vi "CC_Load_Test_REV2.vi"() -> ()   [LabVIEW 2018]
uses:
  <vilib>/Utility/error.llb/DialogType.ctl
  <vilib>/DAQmx/read.llb/DAQmx Read (Analog 1D Wfm NChan NSamp).vi
  <vilib>/Waveform/WDTOps.llb/WDT Get Waveform Time Array DBL.vi
  <vilib>/DAQmx/configure/timing.llb/DAQmx Timing (Sample Clock).vi
  <vilib>/DAQmx/miscellaneous.llb/DAQmx Fill In Error Info.vi
  <resource>/objmgr/daqmx.rc
panel:
  out "Strain Gauges":waveform(dbl)[](graph) caption="Waveform Chart"
  in  "Tab Control":enum32{"Telemetry", "DAQ Settings"}(tab)
  in  "Save 2":bool caption="Save"
  out "Save Path":path caption="Path"
  in  "Test Name":string caption="String"
  in  "Stop 4":bool caption="Stop"
  in  "Strain Tare":bool caption="Reset"
  out "Strain 0":dbl caption="Numeric" format="%#_3e"
  out "Strain 1":dbl caption="Numeric" format="%#_3e"
  out "Strain 2":dbl caption="Numeric" format="%#_3e"
  out "Strain 3":dbl caption="Numeric" format="%#_3e"
  out "Strain 4":dbl caption="Numeric" format="%#_3e"
  out "Strain 5":dbl caption="Numeric" format="%#_3e"
  out "Strain 6":dbl caption="Numeric" format="%#_3e"
  out "Strain 7":dbl caption="Numeric" format="%#_3e"
  out "Strain 8":dbl caption="Numeric" format="%#_3e"
  out "Strain 9":dbl caption="Numeric" format="%#_3e"
  out "Strain 10":dbl caption="Numeric" format="%#_3e"
  out "Strain 11":dbl caption="Numeric" format="%#_3e"
  out "Strain 12":dbl caption="Numeric" format="%#_3e"
  out "Strain 13":dbl caption="Numeric" format="%#_3e"
  out "Strain 14":dbl caption="Numeric" format="%#_3e"
  out "Strain 15":dbl caption="Numeric" format="%#_3e"
  out "LOAD":dbl caption="Numeric"
  out "LOAD 2":dbl caption="Numeric"
  in  "Load Tare":bool caption="Reset"
  in  "Strain Samples Per Loop":i32=100 caption="Numeric"
  out "Strain Output Rate":dbl caption="Numeric"
  in  "Strain Sample Rate":dbl=1000.0 caption="Numeric"
  out "Load Cell Output Rate":dbl caption="Numeric"
  in  "Load Cell Sample Rate":dbl=100.0 caption="Numeric"
  in  "Load Cell Samples Per Loop":i32=10 caption="Numeric"
  out "Load Cell":waveform(dbl)[](graph) caption="Waveform Chart"
  # "Raw"
  # "Tared"
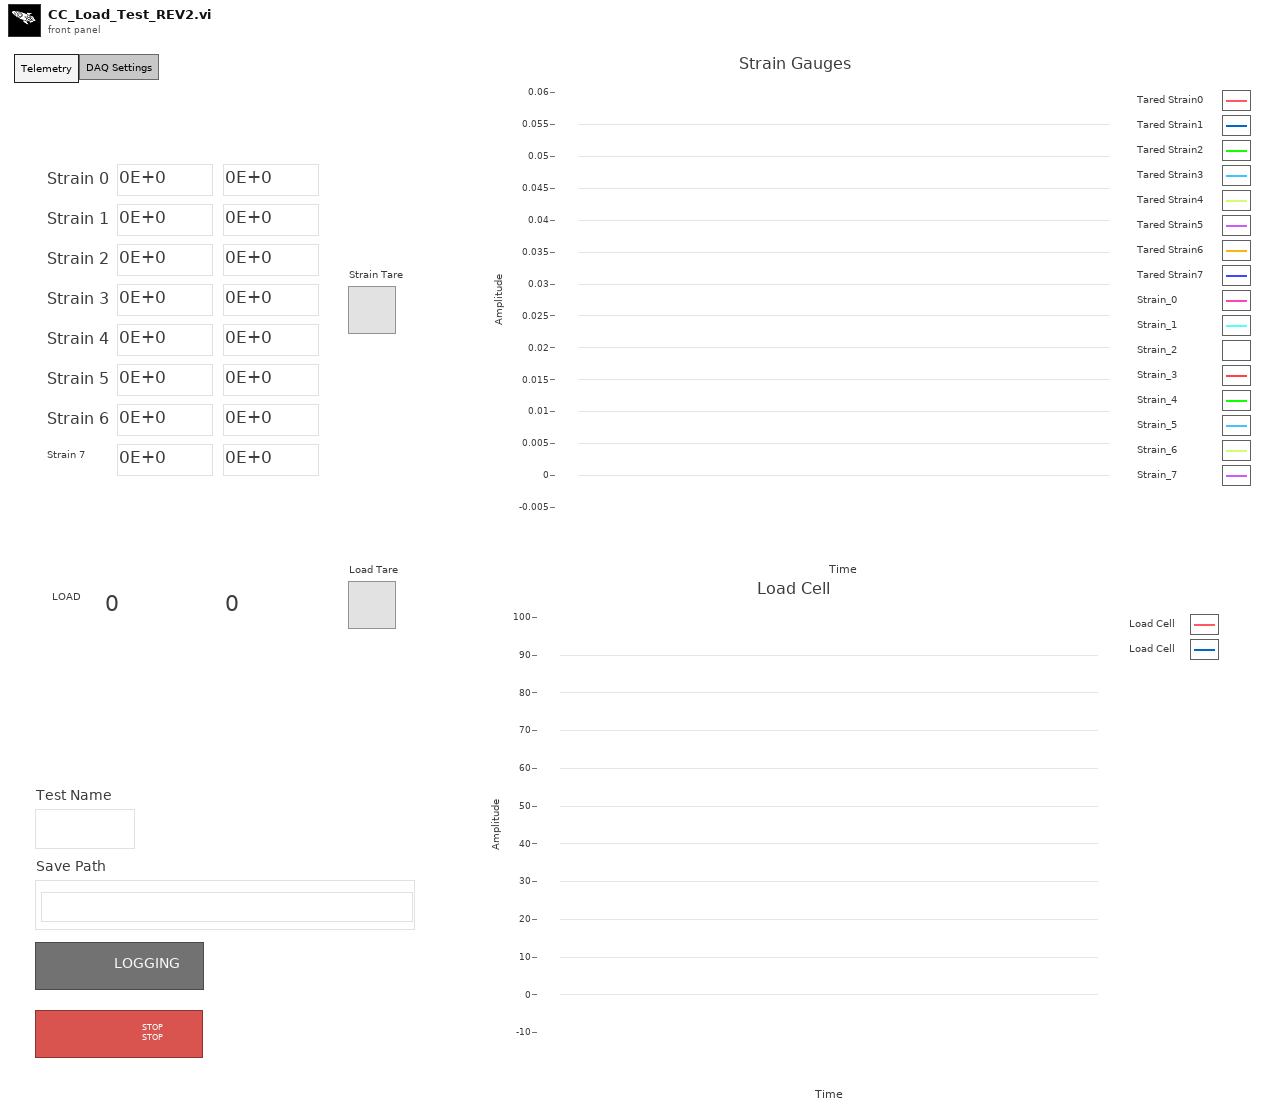
[diagram p1: front panel]
types:
  T1 = typedef "DialogType.ctl" = u16
  T2 = enum16{"open", "open or create", "create or replace", "create", "open (read-only)"}
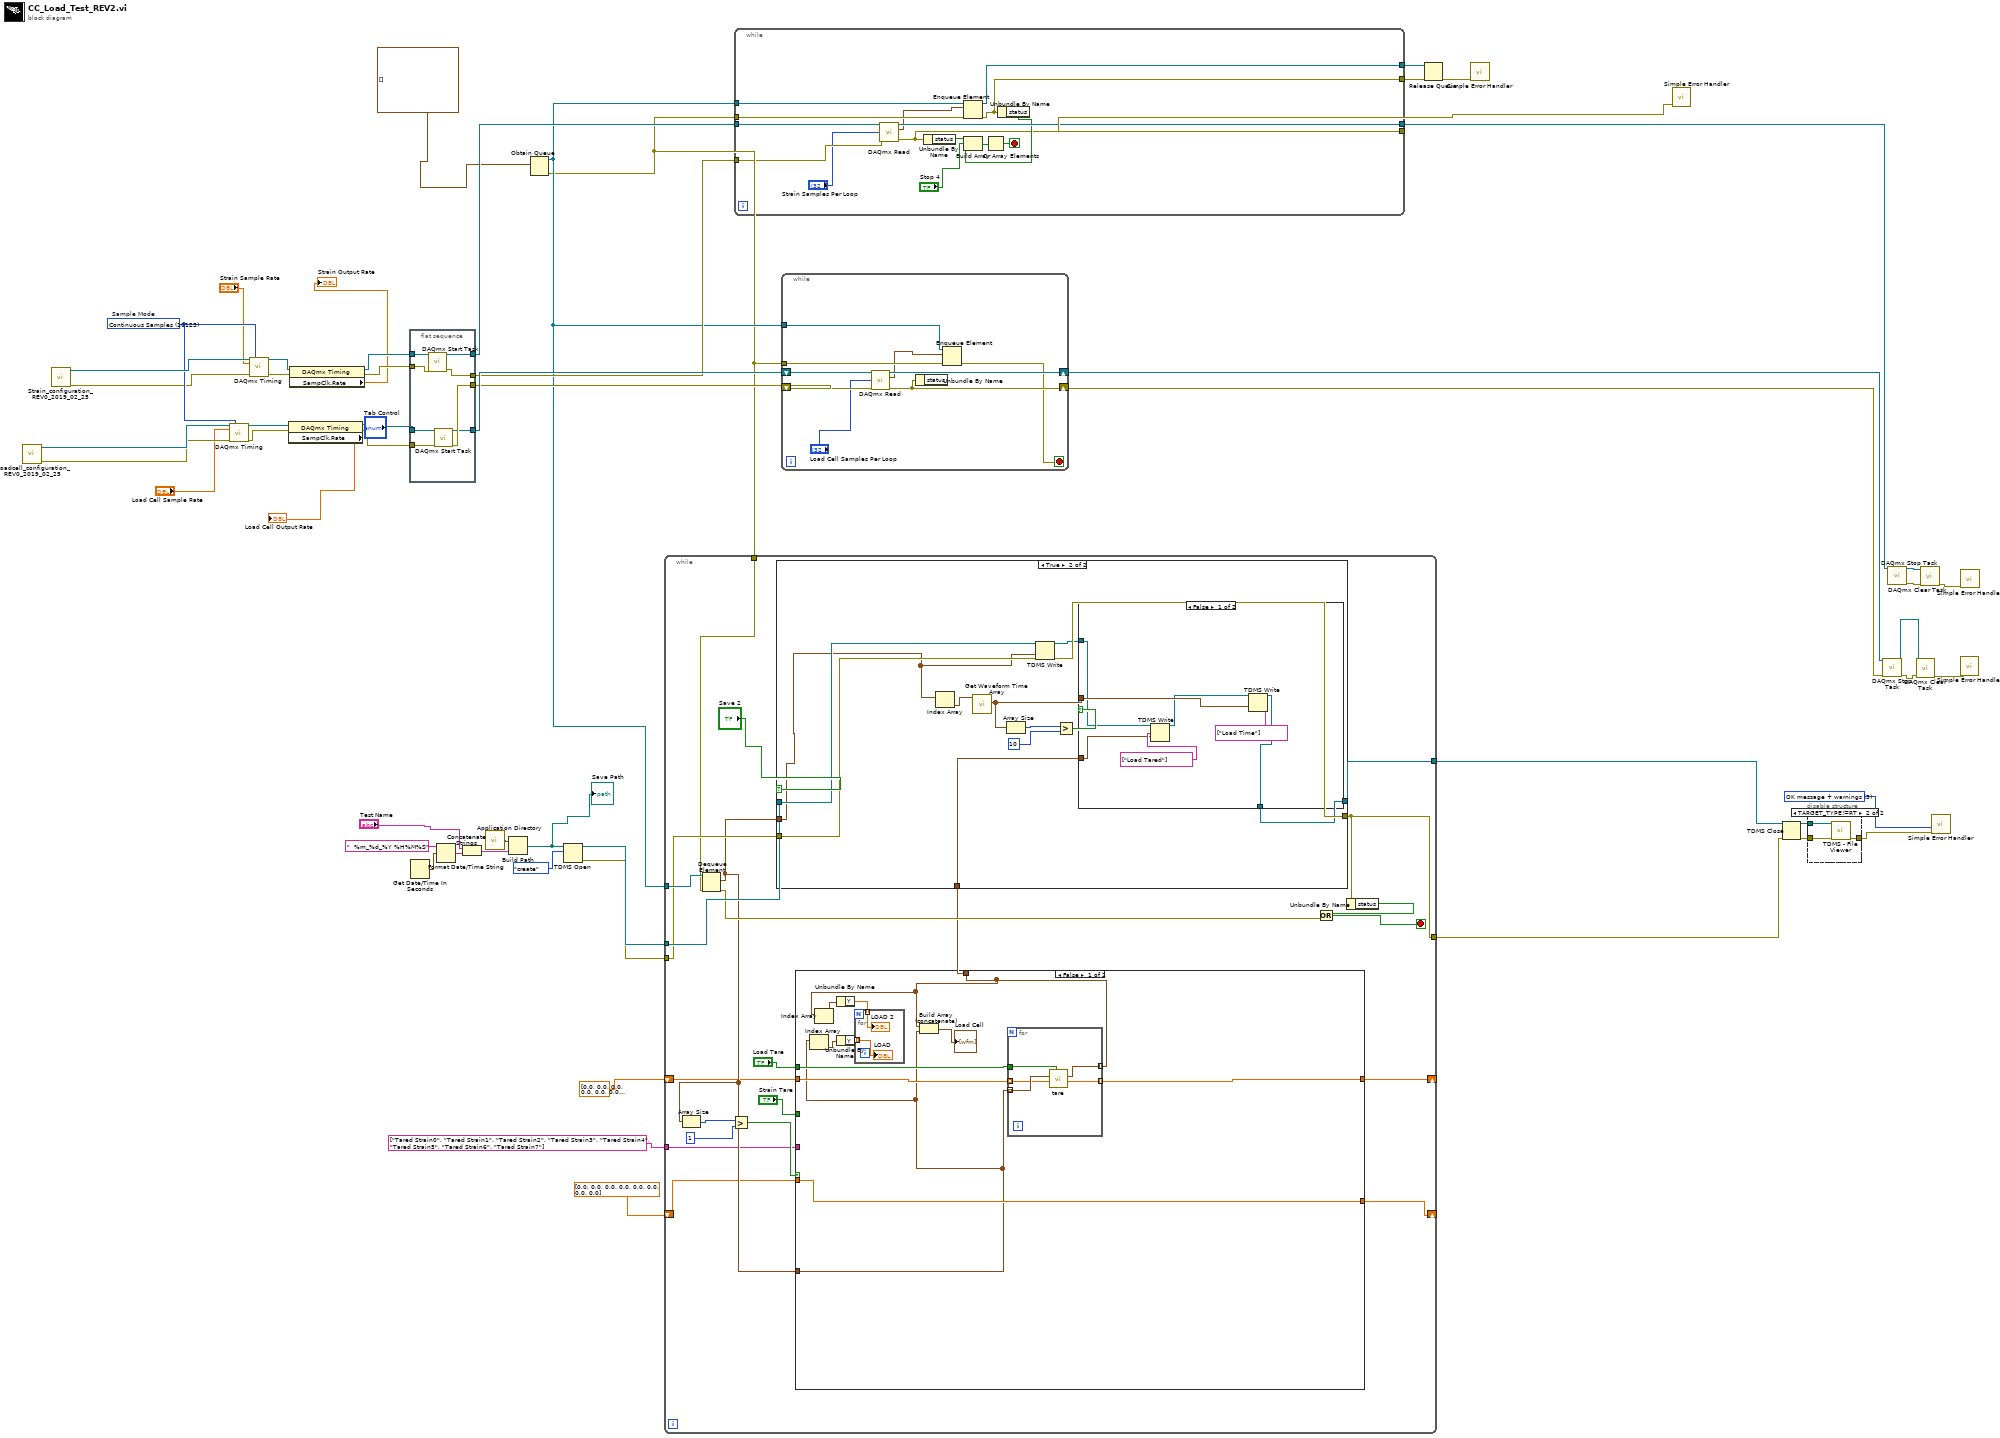
[diagram p0: block diagram]
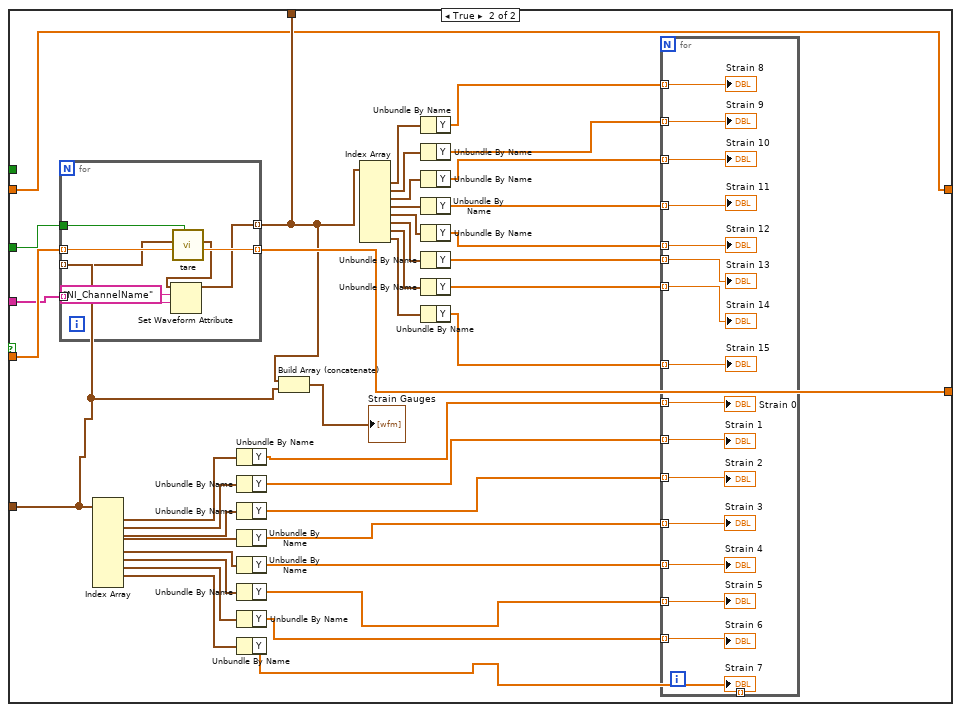
[diagram p3: hidden frame]
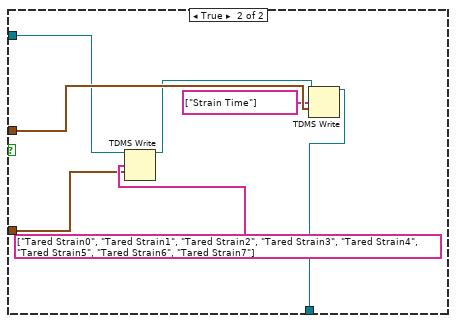
[diagram p5: hidden frame]
diagram:
  w47 = T1 3 items=["no dialog", "OK message", "continue or stop message", "OK message + warnings", "continue/stop + warnings"] ("type of dialog (OK msg:1)")
  w34 = 10123 items=["Finite Samples"=10178, "Continuous Samples"=10123, "Hardware Timed Single Point"=12522]  # Sample Mode
  n1 = call "Loadcell_configuration_REV0_2019_02_25.vi"() -> ("error out"=w24:errorcluster, "task out"=w31:refnum<k21>)  [unwired: 10 in]
  n2 = call "Strain_configuration_REV0_2019_02_25.vi"() -> ("error out"=w25:errorcluster, "task out"=w35:refnum<k21>)  [unwired: 10 in]
  n3 = call-poly <vilib>:"DAQmx Timing.vi"("task/channels in"=w31, "sample mode"=w34, "rate"="Load Cell Sample Rate", "error in"=w24) -> ("task out"=w33:refnum<k21>, "error out"=w32:errorcluster)  [unwired: 10 in]
  n4 = call-poly <vilib>:"DAQmx Timing.vi"("task/channels in"=w35, "sample mode"=w34, "rate"="Strain Sample Rate", "error in"=w25) -> ("task out"=w56:refnum<k21>, "error out"=w55:errorcluster)  [unwired: 10 in]
  n5 = property class="DAQmx Timing"(reference=w33, error in=w32) -> (reference out=w30:refnum<k21>, error out=w22:errorcluster, "SampClk.Rate"=→"Load Cell Output Rate":dbl)
  n6 = property class="DAQmx Timing"(reference=w56, error in=w55) -> (reference out=w50:refnum<k21>, error out=w49:errorcluster, "SampClk.Rate"=→"Strain Output Rate":dbl)
  n7 = flat-sequence {
    tunnel: [w64] -> w54
    tunnel: w50 -> [w63]
    tunnel: w49 -> [w62]
    tunnel: [w61] -> w18
    tunnel: w30 -> [w60]
    tunnel: [w59] -> w17
    tunnel: [w58] -> w20
    tunnel: w22 -> [w57]
    frame #0 {
      n8 = call <vilib>:"DAQmx Start Task.vi"("task/channels in"=w63, "error in"=w62) -> ("task out"=w64:refnum<k21>, "error out"=w61:errorcluster)  [unwired: 12 in]
      n9 = call <vilib>:"DAQmx Start Task.vi"("task/channels in"=w60, "error in"=w57) -> ("task out"=w58:refnum<k21>, "error out"=w59:errorcluster)  [unwired: 12 in]
    }
  }
  n10 = Get Date/Time In Seconds() -> (seconds since 1Jan1904=w40:timestamp)
  n11 = Format Date/Time String(time format string (%c)="  %m_%d_%Y %H%M%S", seconds (now)=w40) -> (date/time string=w37:string)  [unwired: 1 in]
  n12 = Concatenate Strings("Test Name", w37) -> (w36:string)
  n13 = call <vilib>:"Application Directory.vi"() -> ("Application Directory"=w38:path)
  n14 = Build Path(base path=w38, name or relative path=w36) -> (appended path=w5:path)
  "Save Path" <- w5
  n15 = Obtain Queue(element data type=waveform(dbl)[] [] ("data")) -> (queue out=w16:refnum<queue>, error out=w10:errorcluster)  [unwired: 4 in, 1 out]
  n16 = TDMS Open(10:T2."create" ("operation"), 11:w5) -> (0:w41:errorcluster, 3:w46:refnum<k34>)  [unwired: 5 in]
  n17 = while {
    tunnel: w46 -> [w86]
    tunnel: [w85] -> w45
    tunnel: [w82] -> w42
    tunnel: w41 -> [w80]
    tunnel: w16 -> [w81]
    tunnel: w10 -> [w79]
    shift-right: [w70] -> _
    shift-left: dbl[] [0.0, 0.0, 0.0, 0.0, 0.0, 0.0, 0.0, 0.0] ("Shift Registor") -> [w71]
    shift-right: [w67] -> _
    shift-left: dbl[] [0.0, 0.0, 0.0, 0.0, 0.0, 0.0, 0.0, 0.0] ("Shift Registor") -> [w68]
    tunnel: string[] ["Tared Strain0", "Tared Strain1", "Tared Strain2", "Tared Strain3", "Tared Strain4", "Tared Strain5", "Tared Strain6", "Tared Strain7"] ("channel name(s) in (Untitled)") -> [w66]
    stop <- w83 stop-if-true
    n18 = Dequeue Element(queue=w81, error in (no error)=w79) -> (element=w72:waveform(dbl)[], error out=w78:errorcluster)  [unwired: 1 in, 2 out]
    n19 = Array Size(array=w72) -> (size(s)=w75:i32)
    n20 = Greater?(x=w75, y=1) -> (0:w73:bool)
    n21 = case shown="False" w73 {
      tunnel: "Strain Tare" -> [_ w110]
      tunnel: w71 -> [w97 w112]
      tunnel: w72 -> [w89 w109]
      tunnel: [w97 w111] -> w70
      tunnel: [w93 w108] -> w69
      tunnel: w68 -> [w96 w106]
      tunnel: [w95 w106] -> w67
      tunnel: w66 -> [_ w105]
      tunnel: "Load Tare" -> [w90 _]
      frame False {
        n22 = Index Array(array=w89) -> (element=w88:waveform(dbl))  [unwired: 1 in]
        n23 = Unbundle By Name(w88) -> ("Y"=w87:dbl[])
        n24 = for {
          tunnel: w89 -> [w102] mode=indexing
          tunnel: w96 -> [w101] mode=indexing
          tunnel: [w100] -> w95 mode=indexing
          tunnel: [w104] -> w93 mode=indexing
          tunnel: w90 -> [w103]
          n25 = call "tare.vi"("Tare Control"=w103, "Shift Registor"=w101, "Input Waveform"=w102) -> ("Shift Registor Out"=w100:dbl, "output waveform"=w104:waveform(dbl))  [unwired: 7 in]
        }
        n26 = Index Array(array=w93) -> (element=w92:waveform(dbl))  [unwired: 1 in]
        n27 = Unbundle By Name(w92) -> ("Y"=w91:dbl[])
        n28 = for {
          tunnel: w91 -> [w99] mode=indexing
          tunnel: w87 -> [w98] mode=indexing
          "LOAD 2" <- w99
          "LOAD" <- w98
        }
        n29 = Build Array (concatenate)(w93, w89) -> (→"Load Cell":waveform(dbl)[])
      }
      frame True {
        n30 = for {
          tunnel: w109 -> [w165] mode=indexing
          tunnel: w112 -> [w168] mode=indexing
          tunnel: [w167] -> w111 mode=indexing
          tunnel: [w163] -> w108 mode=indexing
          tunnel: w110 -> [w166]
          tunnel: w105 -> [w162] mode=indexing
          n31 = call "tare.vi"("Tare Control"=w166, "Shift Registor"=w168, "Input Waveform"=w165) -> ("Shift Registor Out"=w167:dbl, "output waveform"=w164:waveform(dbl))  [unwired: 7 in]
          n32 = Set Waveform Attribute(5:w162, 6:"NI_ChannelName" ("name"), 7:w164) -> (3:w163:waveform(dbl))  [unwired: 1 in, 2 out]
        }
        n33 = Index Array(array=w109) -> (element #1=w144:waveform(dbl), element #2=w142:waveform(dbl), element #3=w140:waveform(dbl), element #4=w139:waveform(dbl), element #5=w138:waveform(dbl), element #6=w137:waveform(dbl), element #7=w136:waveform(dbl), element #8=w135:waveform(dbl))  [unwired: 9 in, 1 out]
        n34 = Unbundle By Name(w144) -> ("Y"=w143:dbl[])
        n35 = Unbundle By Name(w142) -> ("Y"=w141:dbl[])
        n36 = Unbundle By Name(w140) -> ("Y"=w134:dbl[])
        n37 = Unbundle By Name(w139) -> ("Y"=w133:dbl[])
        n38 = Unbundle By Name(w138) -> ("Y"=w132:dbl[])
        n39 = Unbundle By Name(w137) -> ("Y"=w131:dbl[])
        n40 = Unbundle By Name(w136) -> ("Y"=w130:dbl[])
        n41 = Unbundle By Name(w135) -> ("Y"=w129:dbl[])
        n42 = Build Array (concatenate)(w108, w109) -> (→"Strain Gauges":waveform(dbl)[])
        n43 = Index Array(array=w108) -> (element #1=w128:waveform(dbl), element #2=w127:waveform(dbl), element #3=w126:waveform(dbl), element #4=w125:waveform(dbl), element #5=w124:waveform(dbl), element #6=w123:waveform(dbl), element #7=w122:waveform(dbl), element #8=w121:waveform(dbl))  [unwired: 8 in]
        n44 = Unbundle By Name(w128) -> ("Y"=w120:dbl[])
        n45 = Unbundle By Name(w127) -> ("Y"=w119:dbl[])
        n46 = Unbundle By Name(w126) -> ("Y"=w113:dbl[])
        n47 = Unbundle By Name(w125) -> ("Y"=w118:dbl[])
        n48 = Unbundle By Name(w124) -> ("Y"=w117:dbl[])
        n49 = Unbundle By Name(w123) -> ("Y"=w116:dbl[])
        n50 = Unbundle By Name(w122) -> ("Y"=w115:dbl[])
        n51 = Unbundle By Name(w121) -> ("Y"=w114:dbl[])
        n52 = for {
          tunnel: w143 -> [w160] mode=indexing
          tunnel: w141 -> [w159] mode=indexing
          tunnel: w134 -> [w158] mode=indexing
          tunnel: w133 -> [w157] mode=indexing
          tunnel: w132 -> [w156] mode=indexing
          tunnel: w131 -> [w155] mode=indexing
          tunnel: w130 -> [w154] mode=indexing
          tunnel: w129 -> [w153] mode=indexing
          tunnel: w120 -> [w152] mode=indexing
          tunnel: w119 -> [w151] mode=indexing
          tunnel: w118 -> [w150] mode=indexing
          tunnel: w117 -> [w149] mode=indexing
          tunnel: w116 -> [w148] mode=indexing
          tunnel: w115 -> [w147] mode=indexing
          tunnel: w114 -> [w146] mode=indexing
          tunnel: w113 -> [w145] mode=indexing
          "Strain 0" <- w160
          "Strain 1" <- w159
          "Strain 2" <- w158
          "Strain 3" <- w157
          "Strain 4" <- w156
          "Strain 5" <- w155
          "Strain 6" <- w154
          "Strain 7" <- w153
          "Strain 8" <- w152
          "Strain 9" <- w151
          "Strain 10" <- w145
          "Strain 11" <- w150
          "Strain 12" <- w149
          "Strain 13" <- w148
          "Strain 14" <- w147
          "Strain 15" <- w146
        }
      }
    }
    n53 = case shown="True" "Save 2" {
      tunnel: w86 -> [w169 w180]
      tunnel: [w169 w178] -> w85
      tunnel: [w170 w182] -> w82
      tunnel: w80 -> [w170 w181]
      tunnel: w72 -> [_ w173]
      tunnel: w69 -> [_ w171]
      frame False {
      }
      frame True {
        n54 = Index Array(array=w173) -> (element=w179:waveform(dbl))  [unwired: 1 in]
        n55 = call-poly <vilib>:"Get Waveform Time Array.vi"("waveform in"=w179) -> ("X array"=w177:timestamp[])  [unwired: 9 in, 1 out]
        n56 = Array Size(array=w177) -> (size(s)=w176:i32)
        n57 = TDMS Write(0:w180, 9:w173, 11:w181) -> (4:w172:refnum<k34>, 15:w182:errorcluster)  [unwired: 3 in, 2 out]
        n58 = Greater?(x=w176, y=10) -> (0:w174:bool)
        n59 = case shown="False" w174 {
          tunnel: [w187 w194] -> w178
          tunnel: w177 -> [w188 w196]
          tunnel: w172 -> [w184 w193]
          tunnel: w171 -> [w185 w190]
          frame False {
            n60 = TDMS Write(0:w184, 7:string[] ["Load Tared"] ("channel name(s) in (Untitled)"), 9:w185) -> (4:w183:refnum<k34>)  [unwired: 3 in, 3 out]
            n61 = TDMS Write(0:w183, 7:string[] ["Load Time"] ("channel name(s) in (Untitled)"), 9:w188) -> (4:w187:refnum<k34>)  [unwired: 3 in, 3 out]
          }
          frame True {
            n62 = TDMS Write(0:w193, 7:string[] ["Tared Strain0", "Tared Strain1", "Tared Strain2", "Tared Strain3", "Tared Strain4", "Tared Strain5", "Tared Strain6", "Tared Strain7"] ("channel name(s) in (Untitled)"), 9:w190) -> (4:w192:refnum<k34>)  [unwired: 3 in, 3 out]
            n63 = TDMS Write(0:w192, 7:string[] ["Strain Time"] ("channel name(s) in (Untitled)"), 9:w196) -> (4:w194:refnum<k34>)  [unwired: 3 in, 3 out]
          }
        }
      }
    }
    n64 = Unbundle By Name(w82) -> ("status"=w84:bool)
    n65 = Or(x=w84, y=w78) -> (x .or. y?=w83:bool)
  }
  n66 = while {
    tunnel: w54 -> [w206]
    tunnel: [w211] -> w53
    tunnel: w16 -> [w210]
    tunnel: w18 -> [w205]
    tunnel: w10 -> [w204]
    tunnel: [w202] -> w6
    tunnel: [w200] -> w9
    tunnel: [w199] -> w8
    stop <- w209 stop-if-true
    n67 = call-poly <vilib>:"DAQmx Read.vi"("task/channels in"=w206, "number of samples per channel"="Strain Samples Per Loop", "error in"=w205) -> ("task out"=w211:refnum<k21>, "data"=w197:waveform(dbl)[], "error out"=w202:errorcluster)  [unwired: 10 in]
    n68 = Unbundle By Name(w202) -> ("status"=w208:bool)
    n69 = Enqueue Element(queue=w210, element=w197, error in (no error)=w204) -> (queue out=w200:refnum<queue>, error out=w199:errorcluster)  [unwired: 1 in, 1 out]
    n70 = Unbundle By Name(w199) -> ("status"=w203:bool)
    n71 = Build Array(w208, "Stop 4", w203) -> (w207:bool[])
    n72 = Or Array Elements(Boolean array=w207) -> (logical OR=w209:bool)
  }
  n73 = while {
    shift-right: [w217] -> w19
    shift-left: w20 -> [w219]
    shift-right: [w220] -> w21
    shift-left: w17 -> [w218]
    tunnel: w16 -> [w216]
    tunnel: w10 -> [w215]
    stop <- w213 stop-if-true
    n74 = call-poly <vilib>:"DAQmx Read.vi"("task/channels in"=w219, "number of samples per channel"="Load Cell Samples Per Loop", "error in"=w218) -> ("task out"=w217:refnum<k21>, "data"=w212:waveform(dbl)[], "error out"=w220:errorcluster)  [unwired: 10 in]
    n75 = Unbundle By Name(w220) -> ()  [unwired: 1 out]
    n76 = Enqueue Element(queue=w216, element=w212, error in (no error)=w215) -> (error out=w213:errorcluster)  [unwired: 1 in, 2 out]
  }
  n77 = Release Queue(queue=w9, error in (no error)=w8) -> (error out=w7:errorcluster)  [unwired: 1 in, 2 out]
  n78 = call <vilib>:"Simple Error Handler.vi"("error in (no error)"=w7) -> ()  [unwired: 1 in, 8 out]
  n79 = call <vilib>:"Simple Error Handler.vi"("error in (no error)"=w6) -> ()  [unwired: 4 in, 5 out]
  n80 = TDMS Close(8:w42, 11:w45) -> (0:w43:errorcluster, 3:w44:path)
  n81 = disable-structure shown="TARGET_TYPE!=RT" {
    disable-tunnel: w43 -> [w221 w224]
    disable-tunnel: w44 -> [_ w223]
    disable-tunnel: [w221 w222] -> w28
    frame condition #0 {
    }
    frame condition #1 (active) {
      n82 = call <vilib>:"TDMS - File Viewer.vi"("error in (no error)"=w224, "file path"=w223) -> ("error out"=w222:errorcluster)  [unwired: 5 out]
    }
  }
  n83 = call <vilib>:"DAQmx Stop Task.vi"("task/channels in"=w19, "error in"=w21) -> ("task out"=w23:refnum<k21>, "error out"=w29:errorcluster)  [unwired: 12 in]
  n84 = call <vilib>:"DAQmx Stop Task.vi"("task/channels in"=w53) -> ("task out"=w52:refnum<k21>, "error out"=w51:errorcluster)  [unwired: 13 in]
  n85 = call <vilib>:"DAQmx Clear Task.vi"("task in"=w23, "error in"=w29) -> ("error out"=w26:errorcluster)  [unwired: 13 in]
  n86 = call <vilib>:"DAQmx Clear Task.vi"("task in"=w52, "error in"=w51) -> ("error out"=w27:errorcluster)  [unwired: 13 in]
  n87 = call <vilib>:"Simple Error Handler.vi"("type of dialog (OK msg:1)"=w47, "error in (no error)"=w28) -> ()  [unwired: 1 in, 7 out]
  n88 = call <vilib>:"Simple Error Handler.vi"("error in (no error)"=w26) -> ()  [unwired: 1 in, 8 out]
  n89 = call <vilib>:"Simple Error Handler.vi"("error in (no error)"=w27) -> ()  [unwired: 1 in, 8 out]
